vi "读取基本数据.vi"(8 "error in (no error)":errorcluster caption="错误输入（无错误）", 10 "写入缓冲区":string, 11 "设备选择":refnum<visa-resource-name>) -> (0 "error out":errorcluster caption="错误输出", 2 "read buffer":string, 3 "通道编号输出":u32)   [LabVIEW 2020, in "bas_meas.lvlib"]
uses:
  bas_meas.lvlib
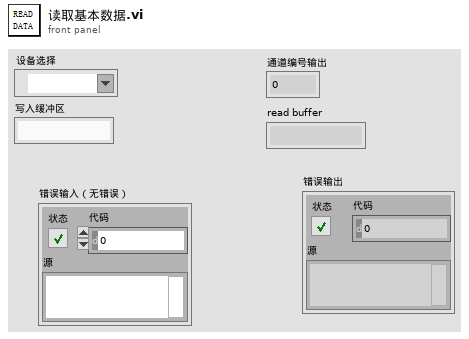
[diagram p1: front panel]
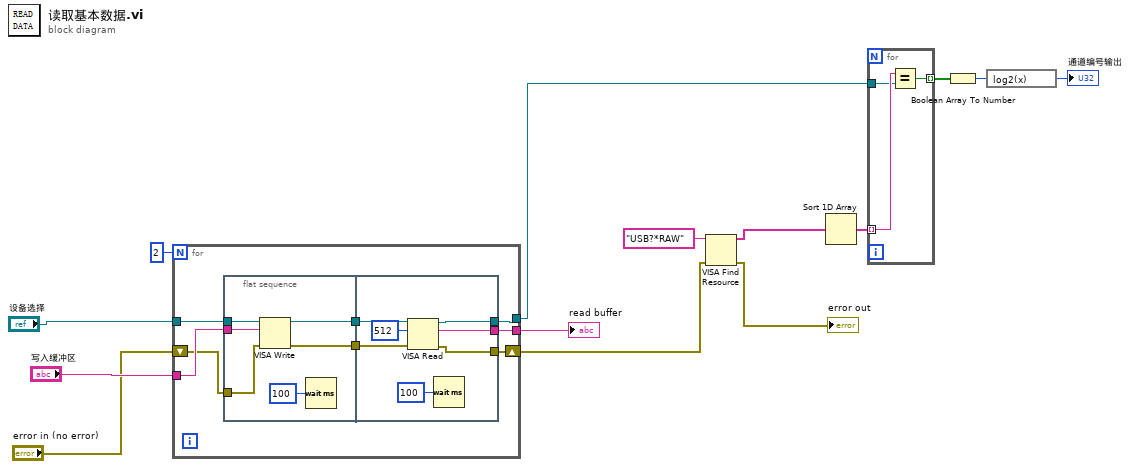
[diagram p0: block diagram]
diagram:
  n1 = for {
    N: 2 -> [_]
    tunnel: "设备选择" -> [w20]
    tunnel: "写入缓冲区" -> [w19]
    tunnel: [w18] -> w12
    shift-right: [w17] -> w4
    shift-left: "error in (no error)" -> [w16]
    tunnel: [w15] -> w1
    n2 = flat-sequence {
      tunnel: w20 -> [w28]
      tunnel: w19 -> [w27]
      tunnel: [w26] -> w22
      tunnel: [w25] -> w21
      tunnel: w16 -> [w23]
      tunnel: w22 -> [w35]
      tunnel: w21 -> [w34]
      tunnel: [w33] -> w18
      tunnel: [w30] -> w17
      tunnel: [w29] -> w15
      frame #0 {
        n3 = VISA Write(VISA resource name=w28, write buffer=w27, error in (no error)=w23) -> (VISA resource name out=w26:refnum<visa-resource-name>, error out=w25:errorcluster)  [unwired: 1 out]
        n4 = Wait (ms)(milliseconds to wait=u32 100 ("等待时间（毫秒）")) -> ()  [unwired: 1 out]
      }
      frame #1 {
        n5 = VISA Read(VISA resource name=w35, byte count=u32 512 ("字节总数"), error in (no error)=w34) -> (VISA resource name out=w29:refnum<visa-resource-name>, read buffer=w33:string, error out=w30:errorcluster)  [unwired: 1 out]
        n6 = Wait (ms)(milliseconds to wait=u32 100 ("等待时间（毫秒）")) -> ()  [unwired: 1 out]
      }
    }
  }
  "read buffer" <- w12
  n7 = VISA Find Resource(8:w4, 11:"USB?*RAW" ("表达式(\"?*\")")) -> (0:→"error out":errorcluster, 3:w10:string[])  [unwired: 1 in, 1 out]
  n8 = Sort 1D Array(array=w10) -> (sorted array=w9:string[])
  n9 = for {
    tunnel: w9 -> [w38] mode=indexing
    tunnel: [w37] -> w8 mode=indexing
    tunnel: w1 -> [w36]
    n10 = Equal?(x=w38, y=w36) -> (x = y?=w37:bool)
  }
  n11 = Boolean Array To Number(Boolean array=w8) -> (number=w7:u32)
  n12 = expression code="log2(x)"(w7) -> (→"通道编号输出":u32)
